vi "Copy from server to public.vi"(9 "Running on Server?":bool, 10 "Path of File relative to EnFlo Data Root":path[](array[path]), 11 "Application in":refnum<vi>) -> (0 "error out":errorcluster, 2 "Problem Files":path[](array[path]), 3 "Relative Paths Out":path[](array[path]))   [LabVIEW 2016]
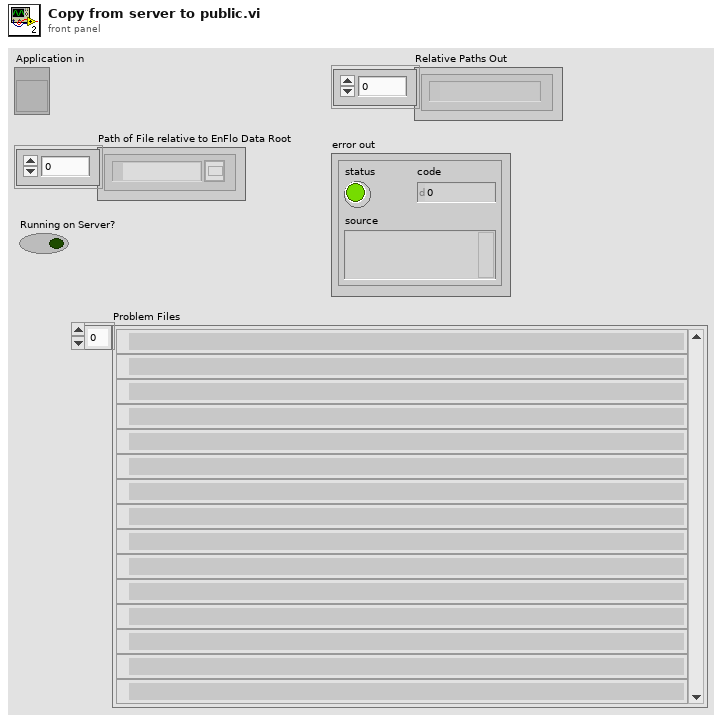
[diagram p1: front panel]
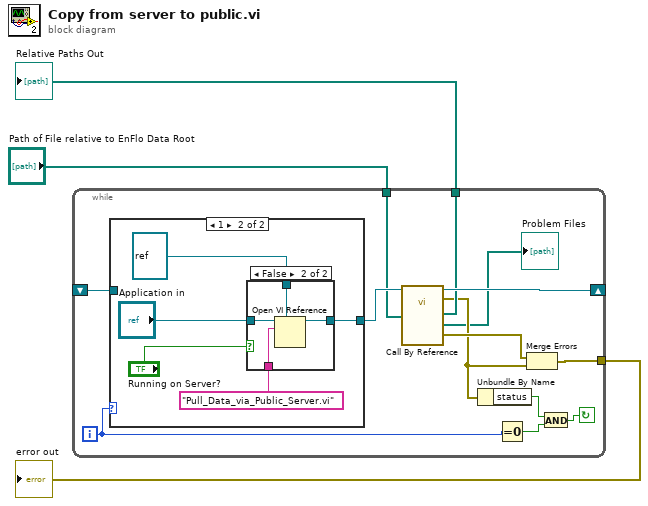
[diagram p0: block diagram]
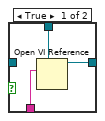
[diagram p3: hidden frame]
diagram:
  n1 = while {
    shift-right: [w14] -> _
    shift-left: _ -> [w16]
    tunnel: "Path of File relative to EnFlo Data Root" -> [w9]
    tunnel: [w8] -> w2
    tunnel: [w5] -> w3
    i -> [w13]
    stop <- w10 continue-if-true
    n2 = case shown="1" w13 {
      tunnel: w16 -> [w17 _]
      tunnel: [w17 w22] -> w15
      frame 0, Default {
      }
      frame 1 {
        n3 = case shown="False" "Running on Server?" {
          tunnel: [w25 w29] -> w22
          tunnel: "Application in" -> [_ w28]
          tunnel: refnum<vi> refnum ("Push Data Server") -> [w24 w27]
          tunnel: "Pull_Data_via_Public_Server.vi" -> [w23 w26]
          frame True {
            n4 = Open VI Reference(type specifier VI Refnum (for type only)=w24, vi path=w23) -> (vi reference=w25:refnum<vi>)  [unwired: 2 in, 3 out]
          }
          frame False {
            n5 = Open VI Reference(type specifier VI Refnum (for type only)=w27, application reference (local)=w28, vi path=w26) -> (vi reference=w29:refnum<vi>)  [unwired: 1 in, 3 out]
          }
        }
      }
    }
    n6 = call-by-ref "?"(reference=w15, "Path of File relative to EnFlo Data Root"=w9) -> (reference out=w14:refnum<vi>, error out=w6:errorcluster, "Relative Paths Out"=w8:path[], "Problem Files"=→"Problem Files":path[], "error out"=w7:errorcluster)  [unwired: 2 in]
    n7 = Unbundle By Name(w6) -> ("status"=w11:bool)
    n8 = Equal To 0?(x=w13) -> (x = 0?=w12:bool)
    n9 = Merge Errors(w7, w6) -> (w5:errorcluster)
    n10 = And(x=w11, y=w12) -> (x .and. y?=w10:bool)
  }
  "error out" <- w3
  "Relative Paths Out" <- w2
